vi "Insight_Laser_Error.vi"(8 "error in (no error)":errorcluster, 11 "telnet connection":T1) -> (0 "error out":errorcluster, 2 "response data":string, 3 "telnet  connection out":T1)   [LabVIEW 2011]
doc: "Insight Photonic Solutions\n\nThis VI sets the Window used to calculate the FFT in Measurement Mode.\n\nver 1.0 - original release"
uses:
  Telnet Session.ctl
  <vilib>/Utility/error.llb/DialogType.ctl
panel:
  out "response data 2":string
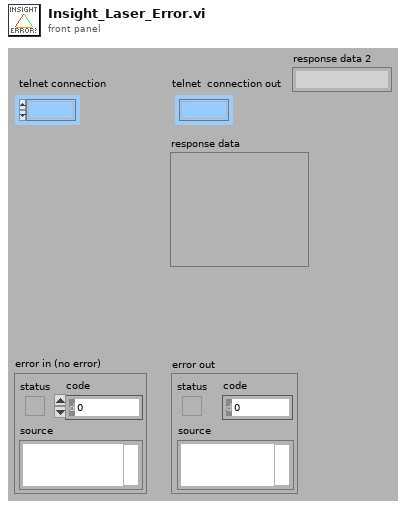
[diagram p1: front panel]
types:
  T1 = typedef "Telnet Session.ctl" = refnum<k1>
  T2 = typedef "DialogType.ctl" = u16
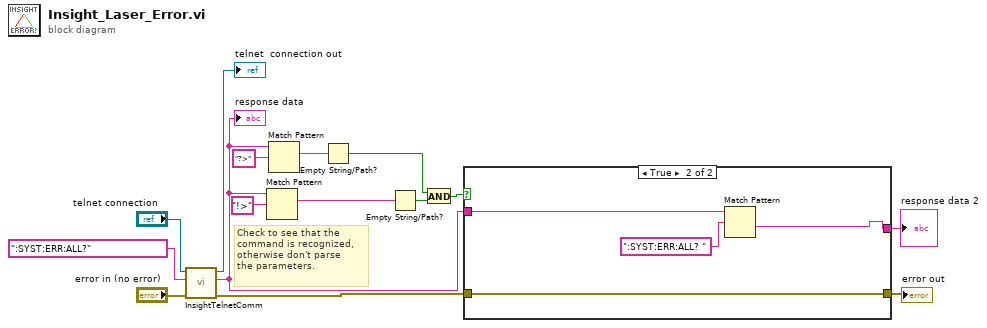
[diagram p0: block diagram]
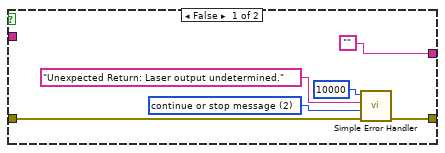
[diagram p2: hidden frame]
diagram:
  # "Check to see that the \ncommand is recognized,\notherwise don't parse \nthe parameters."
  n1 = call "InsightTelnetComm.vi"("error in"="error in (no error)", "write buffer (\"\")"=":SYST:ERR:ALL?" ("String"), "telnet connection"="telnet connection") -> ("error out"=w14:errorcluster, "response data"=w4:string, "telnet  connection out"=→"telnet  connection out":T1)  [unwired: 4 in]
  "response data" <- w4
  n2 = Match Pattern(string=w4, regular expression="!>") -> (match substring=w9:string)  [unwired: 1 in, 3 out]
  n3 = Match Pattern(string=w4, regular expression="?>") -> (match substring=w10:string)  [unwired: 1 in, 3 out]
  n4 = Empty String/Path?(string/path=w10) -> (empty?=w7:bool)
  n5 = Empty String/Path?(string/path=w9) -> (empty?=w6:bool)
  n6 = And(x=w7, y=w6) -> (x .and. y?=w5:bool)
  n7 = case shown="True" w5 {
    tunnel: [w20 w25] -> w15
    tunnel: w14 -> [w21 w25]
    tunnel: w4 -> [_ w23]
    tunnel: ["" w22] -> w1
    frame False {
      w17 = T2 2 items=["no dialog", "OK message", "continue or stop message", "OK message + warnings", "continue/stop + warnings"] ("type of dialog (OK msg:1)")
      n8 = call <vilib>:"Simple Error Handler.vi"("error code (no error:0)"=10000, "error source (\" \")"="Unexpected Return: Laser output undetermined." ("error source (\" \")"), "type of dialog (OK msg:1)"=w17, "error in (no error)"=w21) -> ("error out"=w20:errorcluster)  [unwired: 1 in, 4 out]
    }
    frame True {
      n9 = Match Pattern(string=w23, regular expression=":SYST:ERR:ALL? ") -> (after substring=w22:string)  [unwired: 1 in, 3 out]
    }
  }
  "error out" <- w15
  "response data 2" <- w1
